vi "TurtleLogin.vi"(2 "error in":errorcluster, 3 "Connection Info":T1={"address"="192.168.1.16", "user"="turtlebot", "password"="turtlebot"}) -> (0 "error out":errorcluster, 1 "connection ID out":refnum<k5>)   [LabVIEW 2012]
panel:
  out "passwrd":bool
  out "user":bool
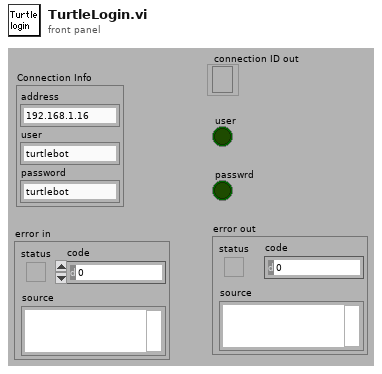
[diagram p1: front panel]
types:
  T1 = cluster{"address":string, "user":string, "password":string}
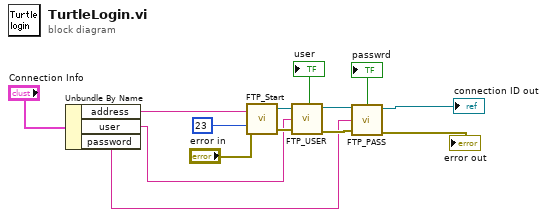
[diagram p0: block diagram]
diagram:
  n1 = Unbundle By Name("Connection Info") -> ("address"=w4:string, "user"=w3:string, "password"=w2:string)
  n2 = call <userlib>:"FTP_Start.vi"("address"=w4, "remote port (21)"=u16 23, "error in (no error)"="error in") -> ("connection ID"=w11:refnum<k5>, "error out"=w10:errorcluster)  [unwired: 1 in, 2 out]
  n3 = call <userlib>:"FTP_USER.vi"("connection ID"=w11, "user"=w3, "error out"=w10) -> ("connection ID out"=w8:refnum<k5>, "Good Reply?"=→"user":bool, "error out 2"=w9:errorcluster)  [unwired: 1 out]
  n4 = call <userlib>:"FTP_PASS.vi"("connection ID"=w8, "password"=w2, "error in"=w9) -> ("connection ID out"=→"connection ID out":refnum<k5>, "Good Reply?"=→"passwrd":bool, "error out"=→"error out":errorcluster)  [unwired: 1 out]
